vi "avoidDisturbAttackerShoot.vi"(1 "CalculatedFollowAttackerPosition":dbl[](array[numeric]), 4 "AttackingOurSelves":bool=TRUE, 5 "Game":refnum<class "Game.lvclass">, 6 "FollowAttackerPosition(FA)":dbl[](array[numeric]), 7 "field_length":i32, 8 "error in (no error)":errorcluster, 9 "AttackerPosition(AT)":dbl[](array[numeric]), 10 "Yball":dbl, 11 "FollowAttackerSkill in":refnum<class "FollowAttackerSkill.lvclass">) -> (0 "error out":errorcluster, 2 "FollowAttackerCorrectedPosition":dbl[](array[numeric]), 3 "FollowAttackerSkill out":refnum<class "FollowAttackerSkill.lvclass">)   [LabVIEW 2023, in "FollowAttackerSkill.lvclass"]
uses:
  FollowAttackerSkill.lvclass
  Game_class/Game.lvclass
  Game_class/Game.lvclass/Game.ctl
  Game_class/Read FieldRef.vi
  Game_class/Read Utilities.lvclass.vi
  Field_class/Field.lvclass
  Utilities_class/Utilities.lvclass
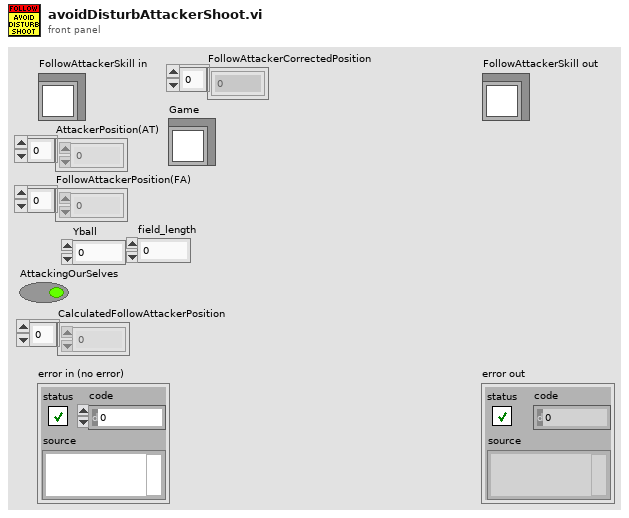
[diagram p1: front panel]
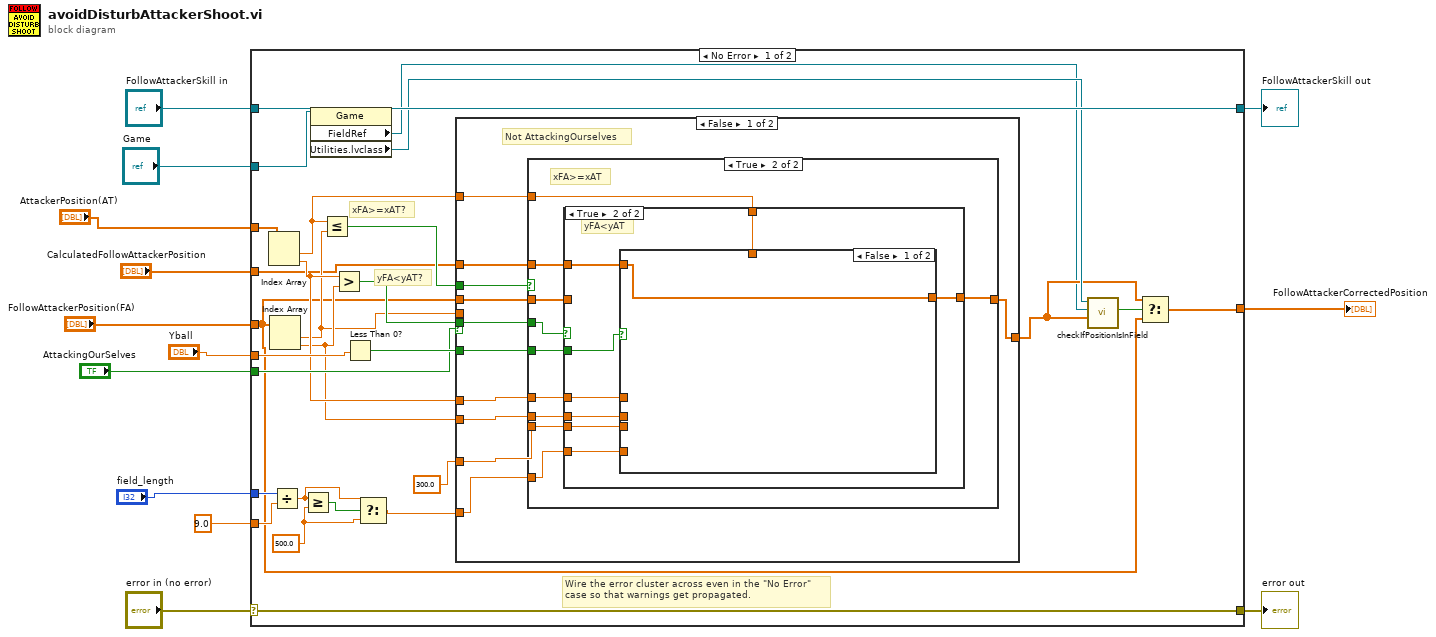
[diagram p0: block diagram]
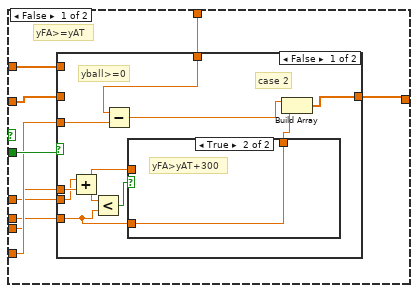
[diagram p3: hidden frame]
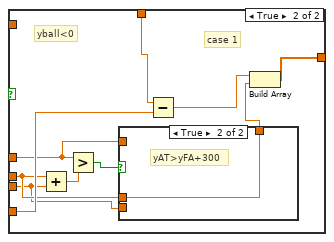
[diagram p6: hidden frame]
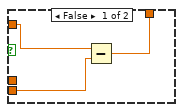
[diagram p7: hidden frame]
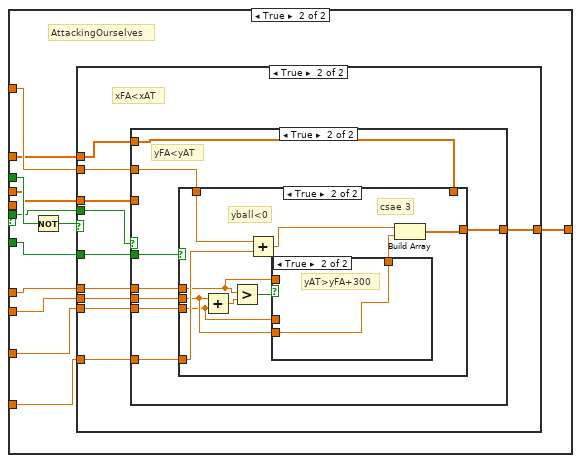
[diagram p8: hidden frame]
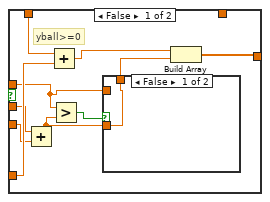
[diagram p11: hidden frame]
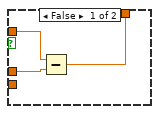
[diagram p14: hidden frame]
diagram:
  n1 = case shown="No Error" "error in (no error)" {
    selector: "error in (no error)" -> [w39 w176]
    tunnel: [w39 w176] -> w12
    tunnel: [w40 w175] -> w10
    tunnel: "FollowAttackerSkill in" -> [w40 w175]
    tunnel: "AttackingOurSelves" -> [w31 _]
    tunnel: "FollowAttackerPosition(FA)" -> [w21 _]
    tunnel: "AttackerPosition(AT)" -> [w38 _]
    tunnel: "Yball" -> [w37 _]
    tunnel: "field_length" -> [w36 _]
    tunnel: 9.0 -> [w35 _]
    tunnel: "Game" -> [w25 _]
    tunnel: [w20 _] -> w2
    tunnel: "CalculatedFollowAttackerPosition" -> [w19 _]
    frame No Error {
      w16 = 500.0 ("element")
      # "yFA<yAT?"
      # "xFA>=xAT?"
      # "Wire the error cluster across even in the \"No Error\"\ncase so that warnings get propagated."
      n2 = Index Array(array=w38) -> (element #1=w30:dbl, element #2=w29:dbl)  [unwired: 2 in]
      n3 = Index Array(array=w21) -> (element #1=w26:dbl, element #2=w27:dbl)  [unwired: 2 in]
      n4 = Divide(x=w36, y=w35) -> (x/y=w17:dbl)
      n5 = Greater Or Equal?(x=w17, y=w16) -> (x >= y?=w18:bool)
      n6 = property class="Game"(reference=w25) -> ("FieldRef"=w14:refnum<class "Field.lvclass">, "Utilities.lvclass"=w24:refnum<class "Utilities.lvclass">)  [unwired: 1 in, 2 out]
      n7 = Less Or Equal?(x=w30, y=w26) -> (x <= y?=w34:bool)
      n8 = Greater?(x=w29, y=w27) -> (0:w33:bool)
      n9 = Less Than 0?(x=w37) -> (x < 0?=w32:bool)
      n10 = Select(t=w17, s=w18, f=w16) -> (s? t:f=w15:dbl)
      n11 = case shown="False" w31 {
        tunnel: w15 -> [w51 w113]
        tunnel: w34 -> [w50 w118]
        tunnel: w33 -> [w49 w117]
        tunnel: w32 -> [w48 w116]
        tunnel: w30 -> [w47 w114]
        tunnel: w29 -> [w46 w110]
        tunnel: 300.0 -> [w45 w112]
        tunnel: w27 -> [w44 w111]
        tunnel: w21 -> [w43 w115]
        tunnel: w26 -> [_ _]
        tunnel: [w42 w109] -> w22
        tunnel: w19 -> [w41 w108]
        frame False {
          # "Not AttackingOurselves"
          n12 = case shown="True" w50 {
            tunnel: w51 -> [_ w59]
            tunnel: w49 -> [_ w62]
            tunnel: w48 -> [_ w61]
            tunnel: w47 -> [_ w60]
            tunnel: w46 -> [_ w58]
            tunnel: w45 -> [_ w57]
            tunnel: w44 -> [_ w56]
            tunnel: w43 -> [_ w55]
            tunnel: [w52 w54] -> w42
            tunnel: w41 -> [w52 w53]
            frame False {
            }
            frame True {
              # "xFA>=xAT"
              n13 = case shown="True" w62 {
                tunnel: w61 -> [w71 w92]
                tunnel: w60 -> [w70 w91]
                tunnel: w59 -> [w69 w90]
                tunnel: w58 -> [w67 w89]
                tunnel: w57 -> [w68 w88]
                tunnel: w56 -> [w66 w87]
                tunnel: w55 -> [w65 _]
                tunnel: [w64 w86] -> w54
                tunnel: w53 -> [w63 w85]
                frame False {
                  # "yFA>=yAT"
                  n14 = case shown="False" w71 {
                    tunnel: w70 -> [w81 _]
                    tunnel: w69 -> [w80 _]
                    tunnel: w68 -> [w79 _]
                    tunnel: w67 -> [w78 _]
                    tunnel: w66 -> [w76 _]
                    tunnel: [w72 w84] -> w64
                    tunnel: w65 -> [_ _]
                    tunnel: w63 -> [_ w84]
                    frame False {
                      # "case 2"
                      # "yball>=0"
                      n15 = Add(x=w78, y=w79) -> (x+y=w75:dbl)
                      n16 = Less?(x=w75, y=w76) -> (x < y?=w77:bool)
                      n17 = Subtract(x=w81, y=w80) -> (x-y=w74:dbl)
                      n18 = case shown="True" w77 {
                        tunnel: [w82 w83] -> w73
                        tunnel: w76 -> [_ w83]
                        tunnel: w75 -> [w82 _]
                        frame False {
                        }
                        frame True {
                          # "yFA>yAT+300"
                        }
                      }
                      n19 = Build Array(w74, w73) -> (w72:dbl[])
                    }
                    frame True {
                    }
                  }
                }
                frame True {
                  # "yFA<yAT"
                  n20 = case shown="False" w92 {
                    tunnel: w91 -> [_ w103]
                    tunnel: w90 -> [_ w102]
                    tunnel: w89 -> [_ w97]
                    tunnel: w88 -> [_ w98]
                    tunnel: w87 -> [_ w99]
                    tunnel: [w93 w94] -> w86
                    tunnel: w85 -> [w93 _]
                    frame False {
                    }
                    frame True {
                      # "case 1"
                      # "yball<0"
                      n21 = Add(x=w99, y=w98) -> (x+y=w100:dbl)
                      n22 = Greater?(x=w97, y=w100) -> (0:w101:bool)
                      n23 = case shown="True" w101 {
                        tunnel: [w104 w107] -> w95
                        tunnel: w99 -> [_ w107]
                        tunnel: w98 -> [w106 _]
                        tunnel: w97 -> [w105 _]
                        frame False {
                          n24 = Subtract(x=w105, y=w106) -> (x-y=w104:dbl)
                        }
                        frame True {
                          # "yAT>yFA+300"
                        }
                      }
                      n25 = Subtract(x=w103, y=w102) -> (x-y=w96:dbl)
                      n26 = Build Array(w96, w95) -> (w94:dbl[])
                    }
                  }
                }
              }
            }
          }
        }
        frame True {
          # "AttackingOurselves"
          n27 = Not(x=w118) -> (.not. x?=w119:bool)
          n28 = case shown="True" w119 {
            tunnel: w117 -> [_ w130]
            tunnel: w116 -> [_ w129]
            tunnel: w115 -> [_ w128]
            tunnel: w114 -> [_ w127]
            tunnel: w113 -> [_ w126]
            tunnel: w112 -> [_ w125]
            tunnel: w111 -> [_ w124]
            tunnel: w110 -> [_ w123]
            tunnel: [w120 w122] -> w109
            tunnel: w108 -> [w120 w121]
            frame False {
            }
            frame True {
              # "xFA<xAT"
              n29 = case shown="True" w130 {
                tunnel: w129 -> [w138 w159]
                tunnel: w128 -> [_ _]
                tunnel: w127 -> [w135 w158]
                tunnel: w126 -> [w136 w157]
                tunnel: w125 -> [w134 w156]
                tunnel: w124 -> [w132 w155]
                tunnel: w123 -> [w133 w154]
                tunnel: [w137 w153] -> w122
                tunnel: w121 -> [w131 w152]
                frame False {
                  # "yFA>=yAT"
                  n30 = case shown="True" w138 {
                    tunnel: [w145 w151] -> w137
                    tunnel: w136 -> [w148 _]
                    tunnel: w135 -> [w147 _]
                    tunnel: w134 -> [w144 _]
                    tunnel: w133 -> [w143 _]
                    tunnel: w132 -> [w140 _]
                    tunnel: w131 -> [_ w151]
                    frame False {
                      # "yball>=0"
                      n31 = Add(x=w143, y=w144) -> (x+y=w139:dbl)
                      n32 = Add(x=w147, y=w148) -> (x+y=w146:dbl)
                      n33 = Greater?(x=w140, y=w139) -> (0:w142:bool)
                      n34 = case shown="False" w142 {
                        tunnel: [w149 w150] -> w141
                        tunnel: w140 -> [_ w150]
                        tunnel: w139 -> [w149 _]
                        frame False {
                        }
                        frame True {
                          # "yFA>yAT+300"
                        }
                      }
                      n35 = Build Array(w146, w141) -> (w145:dbl[])
                    }
                    frame True {
                    }
                  }
                }
                frame True {
                  # "yFA<yAT"
                  n36 = case shown="True" w159 {
                    tunnel: [w160 w166] -> w153
                    tunnel: w158 -> [_ w170]
                    tunnel: w157 -> [_ w169]
                    tunnel: w156 -> [_ w162]
                    tunnel: w155 -> [_ w163]
                    tunnel: w154 -> [_ w161]
                    tunnel: w152 -> [w160 _]
                    frame False {
                    }
                    frame True {
                      # "csae 3"
                      # "yball<0"
                      n37 = Add(x=w163, y=w162) -> (x+y=w167:dbl)
                      n38 = Greater?(x=w161, y=w167) -> (0:w168:bool)
                      n39 = Add(x=w170, y=w169) -> (x+y=w165:dbl)
                      n40 = case shown="True" w168 {
                        tunnel: [w171 w174] -> w164
                        tunnel: w163 -> [_ w174]
                        tunnel: w162 -> [w173 _]
                        tunnel: w161 -> [w172 _]
                        frame False {
                          n41 = Subtract(x=w172, y=w173) -> (x-y=w171:dbl)
                        }
                        frame True {
                          # "yAT>yFA+300"
                        }
                      }
                      n42 = Build Array(w165, w164) -> (w166:dbl[])
                    }
                  }
                }
              }
            }
          }
        }
      }
      n43 = call "checkIfPositionIsInField.vi"("Position"=w22, "FieldRef"=w14, "Utilities in"=w24) -> ("Position Is In Field?"=w23:bool)  [unwired: 4 in, 4 out]
      n44 = Select(t=w22, s=w23, f=w21) -> (s? t:f=w20:dbl[])
    }
    frame Error {
    }
  }
  "error out" <- w12
  "FollowAttackerSkill out" <- w10
  "FollowAttackerCorrectedPosition" <- w2
